vi "Settings Dialog.vi"(8 "error in (no error)":errorcluster, 11 "Settings in":T1) -> (0 "error out":errorcluster, 1 "Cancelled?":bool=TRUE, 2 "UI Refresh Needed?":bool, 3 "Settings out":T5={"Hardware Configuration"={"Analog Out array"=[], "Initialize Flag"=FALSE, "Saftey Table Display"=refnum, "Torque&Force"=[], "Calibration Data"=[], "2D"=[], "Analog In Task"="", "Digital In Task"="", "Analog Out Task"="", "Digital Out Task"="", "Digital Out Array"=[], "Current Cycle Count"=refnum, "Cycle Count"=0, "Headers"=[], "Sweep Interval"=0, "Delay"=0, "TestConfigDisplay"=refnum, "50psi Conversion"=[], "1245N15 Conversion"=[], "MX06F Conversion"=[], "# of Test Cycles"=0, "60psi Conversion"=[], "100psi Conversion"=[], "200psi Conversion"=[], "1000psi Conversion"=[], "2000psi Conversion"=[], "5000psi Conversion"=[], "MX09F Conversion"=[], "MX19F Conversion"=[]}, "Logging Configuration"={"Log File Base Path"=path "C:/Users/jpassiak/Documents/LabVIEW Data/Logged Data.tdms", "TDMS File Reference"=refnum, "Samples to Save"=0, "Trigger - Time"=0, "Trigger - Threshold"=0.0, "Trigger - Channel"=0, "Enable Time Trigger"=FALSE, "Enable Threshold Trigger"=FALSE, "Always Log"=FALSE}, "Configuration Data"={}})   [LabVIEW 2026, in "Settings.lvlib"]
doc: "Dialog for selecting user specified settings."
uses:
  Settings.lvlib
  <vilib>/Utility/xml.llb/Write to XML File(string).vi
  Acquisition/Hardware Configuration.ctl
  Acquisition/Acquisition.lvlib
  Logging/Logging Configuration.ctl
  Logging/Logging.lvlib
  Settings.ctl
  controls/Test Config Data.ctl
panel:
  in  "Log when triggered":bool
  in  "Trigger Channel":u32
  in  "Samples to Log":u32=500 min=1
  in  "Trigger Threshold (V)":dbl=2.0
  in  "Trigger Time (min)":u32=1
  in  "Enable Threshold Trigger (V):":bool
  in  "Enable Time Trigger (min):":bool
  in  "Always Log":bool
  in  "Sample Rate":dbl=1000.0
  in  "Minimum Input":dbl=-10.0
  in  "Maximum Input":dbl=10.0
  in  "DAQmx Channel":tag="Dev1/ai0"
  in  "Log File Path":path
  in  "Cancel Button":bool
  in  "OK Button":bool
  # "Acquisition"
  # "Non visible portion of dialog (needed for connector pane)."
  # "Trigger"
  # "Logging"
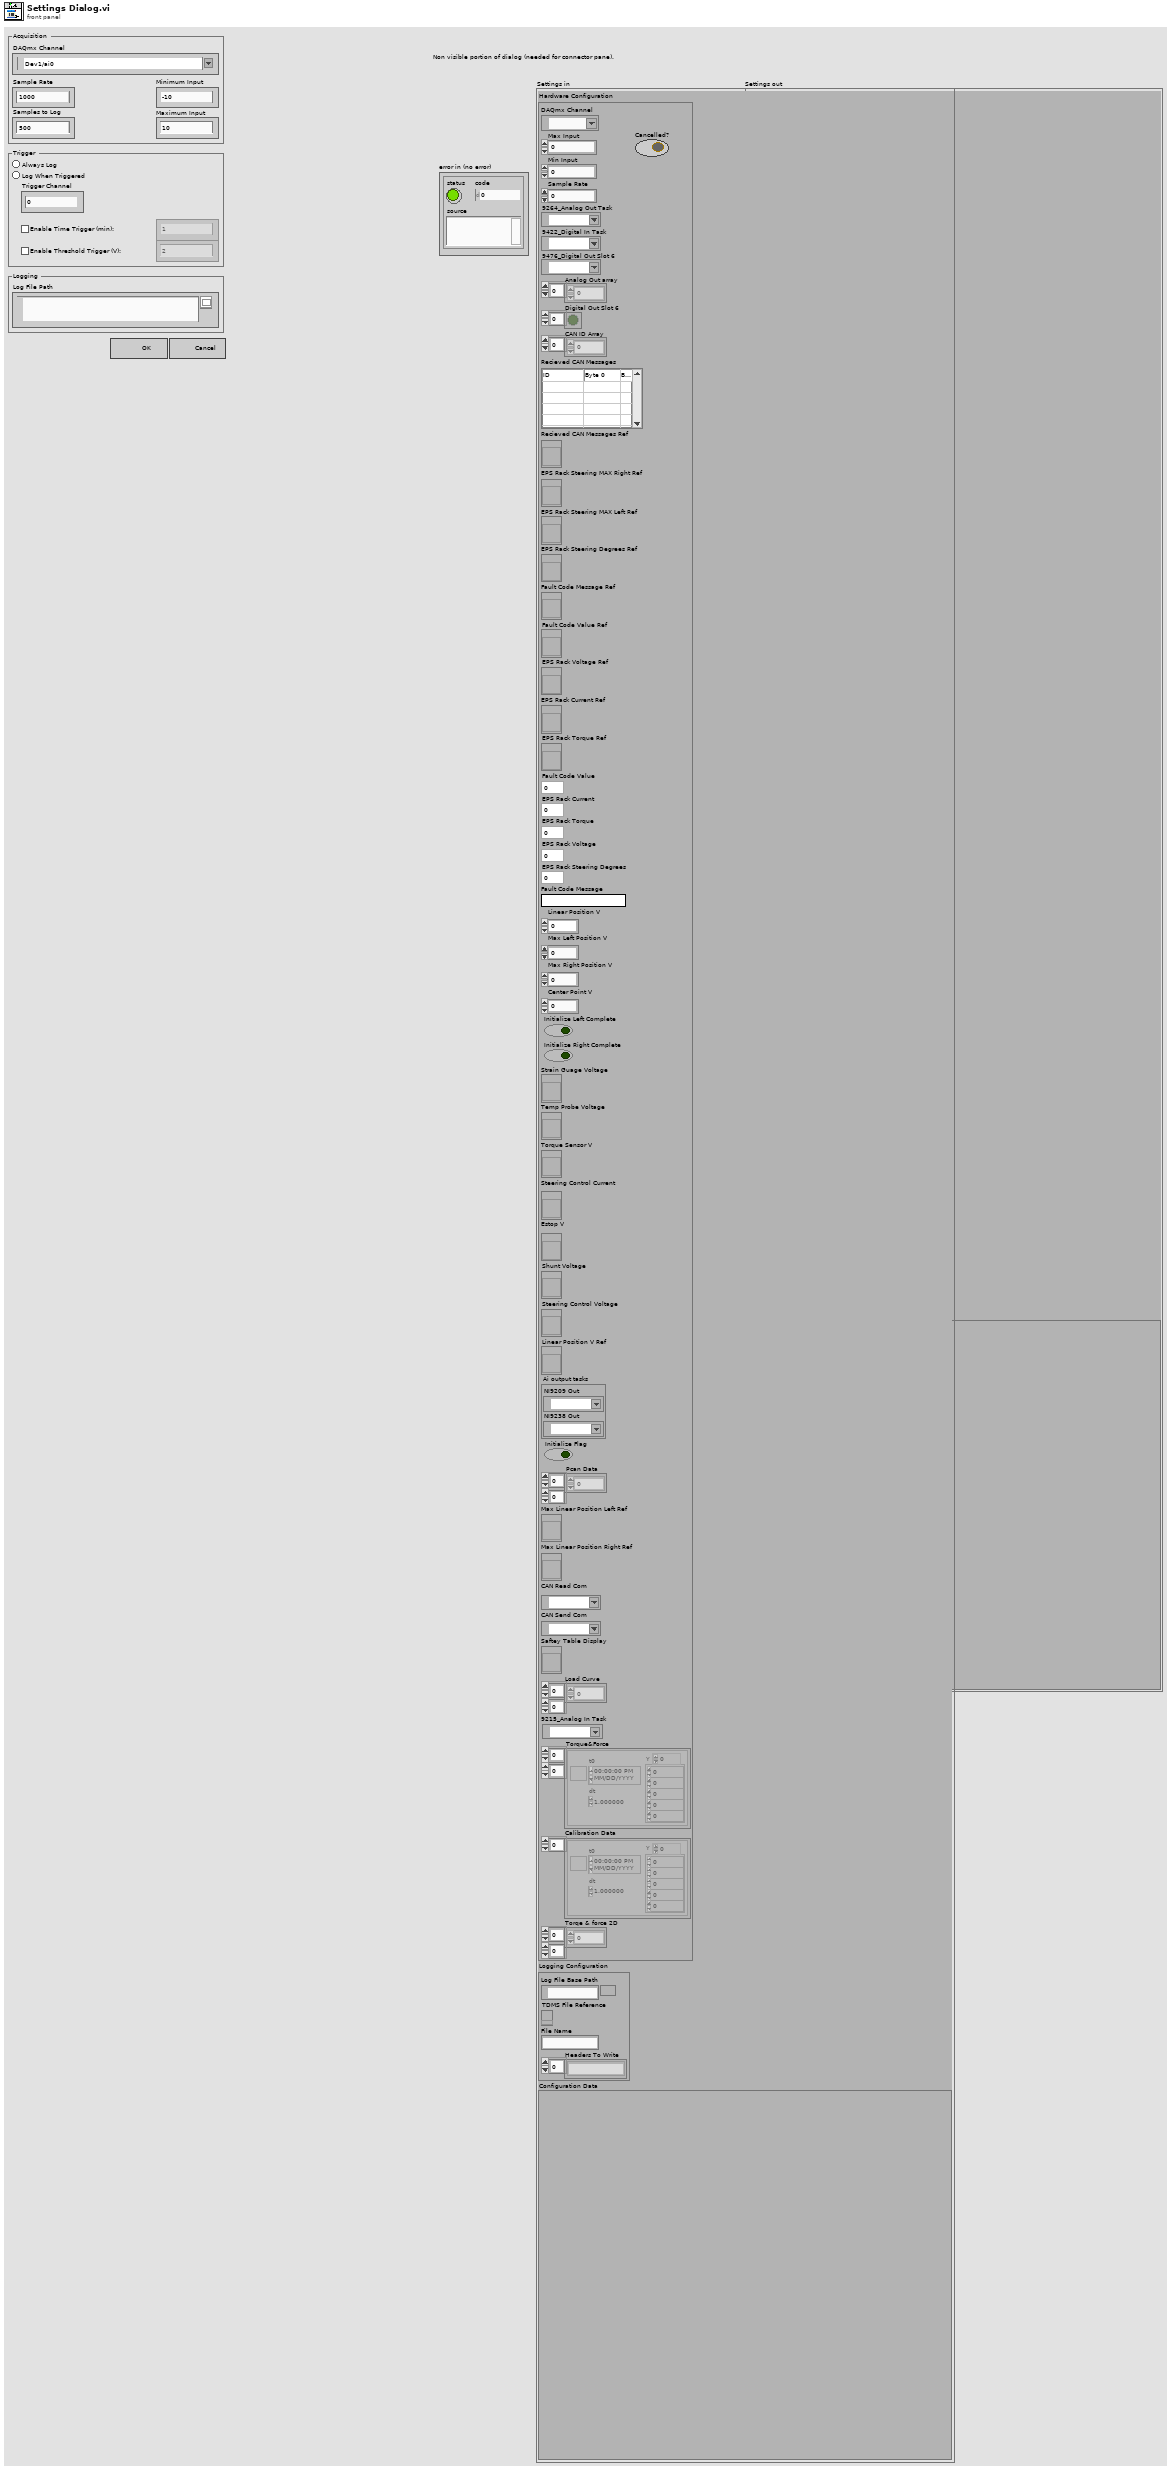
[diagram p1: front panel]
types:
  T1 = typedef "Settings.lvlib/Settings.ctl" = cluster{"Hardware Configuration":T2, "Logging Configuration":T3, "Configuration Data":T4}
  T2 = typedef "Acquisition.lvlib/Hardware Configuration.ctl" = cluster{"DAQmx Channel":tag, "Max Input":dbl, "Min Input":dbl, "Sample Rate":dbl, "9264_Analog Out Task":refnum<k21>, "9422_Digital In Task":refnum<k21>, "9476_Digital Out Slot 6":refnum<k21>, "Analog Out array":dbl[], "Digital Out Slot 6":bool[], "CAN ID Array":u32[], "Recieved CAN Messages ":string[][], "Recieved CAN Messages Ref":refnum<vi>, "EPS Rack Steering MAX Right Ref":refnum<vi>, "EPS Rack Steering MAX Left Ref":refnum<vi>, "EPS Rack Steering Degrees Ref":refnum<vi>, "Fault Code Message Ref":refnum<vi>, "Fault Code Value Ref":refnum<vi>, "EPS Rack Voltage Ref":refnum<vi>, "EPS Rack Current Ref":refnum<vi>, "EPS Rack Torque Ref":refnum<vi>, "Fault Code Value":dbl, "EPS Rack Current":dbl, "EPS Rack Torque":dbl, "EPS Rack Voltage":dbl, "EPS Rack Steering Degrees":dbl, "Fault Code Message":string, "Linear Position V":dbl, "Max Left Position V":dbl, "Max Right Position V":dbl, "Center Point V":dbl, "Initialize Left Complete":bool, "Initialize Right Complete":bool, "Strain Guage Voltage":refnum<vi>, "Temp Probe Voltage":refnum<vi>, "Torque Sensor V":refnum<vi>, "Steering Control Current":refnum<vi>, "Estop V":refnum<vi>, "Shunt Voltage":refnum<vi>, "Steering Control Voltage":refnum<vi>, "Linear Position V Ref":refnum<vi>, "Ai output tasks":cluster{"NI9209 Out":refnum<k21>, "NI9238 Out":refnum<k21>}, "Initialize Flag":bool, "Pcan Data":dbl[][], "Max Linear Position Left Ref":refnum<vi>, "Max Linear Position Right Ref":refnum<vi>, "CAN Read Com":refnum<k21>, "CAN Send Com":refnum<k21>, "Saftey Table Display":refnum<vi>, "Load Curve":dbl[][], "9215_Analog In Task":refnum<k21>, "Torque&Force":waveform(dbl)[][], "Calibration Data":waveform(dbl)[], "Torqe & force 2D":dbl[][]}
  T3 = typedef "Logging.lvlib/Logging Configuration.ctl" = cluster{"Log File Base Path":path, "TDMS File Reference":refnum<k34>, "File Name":string, "Headers To Write":string[]}
  T4 = typedef "Test Config Data.ctl" = cluster{}
  T5 = typedef "Settings.lvlib/Settings.ctl" = cluster{"Hardware Configuration":T6, "Logging Configuration":T7, "Configuration Data":T4}
  T6 = typedef "Acquisition.lvlib/Hardware Configuration.ctl" = cluster{"Analog Out array":dbl[], "Initialize Flag":bool, "Saftey Table Display":refnum<vi>, "Torque&Force":waveform(dbl)[][], "Calibration Data":waveform(dbl)[], "2D":dbl[][], "Analog In Task":refnum<k21>, "Digital In Task":refnum<k21>, "Analog Out Task":refnum<k21>, "Digital Out Task":refnum<k21>, "Digital Out Array":bool[], "Current Cycle Count":refnum<vi>, "Cycle Count":u64, "Headers":string[], "Sweep Interval":u64, "Delay":u64, "TestConfigDisplay":refnum<vi>, "50psi Conversion":dbl[], "1245N15 Conversion":dbl[], "MX06F Conversion":dbl[], "# of Test Cycles":u64, "60psi Conversion":dbl[], "100psi Conversion":dbl[], "200psi Conversion":dbl[], "1000psi Conversion":dbl[], "2000psi Conversion":dbl[], "5000psi Conversion":dbl[], "MX09F Conversion":dbl[], "MX19F Conversion":dbl[]}
  T7 = typedef "Logging.lvlib/Logging Configuration.ctl" = cluster{"Log File Base Path":path, "TDMS File Reference":refnum<k34>, "Samples to Save":u32, "Trigger - Time":u32, "Trigger - Threshold":dbl, "Trigger - Channel":u32, "Enable Time Trigger":bool, "Enable Threshold Trigger":bool, "Always Log":bool}
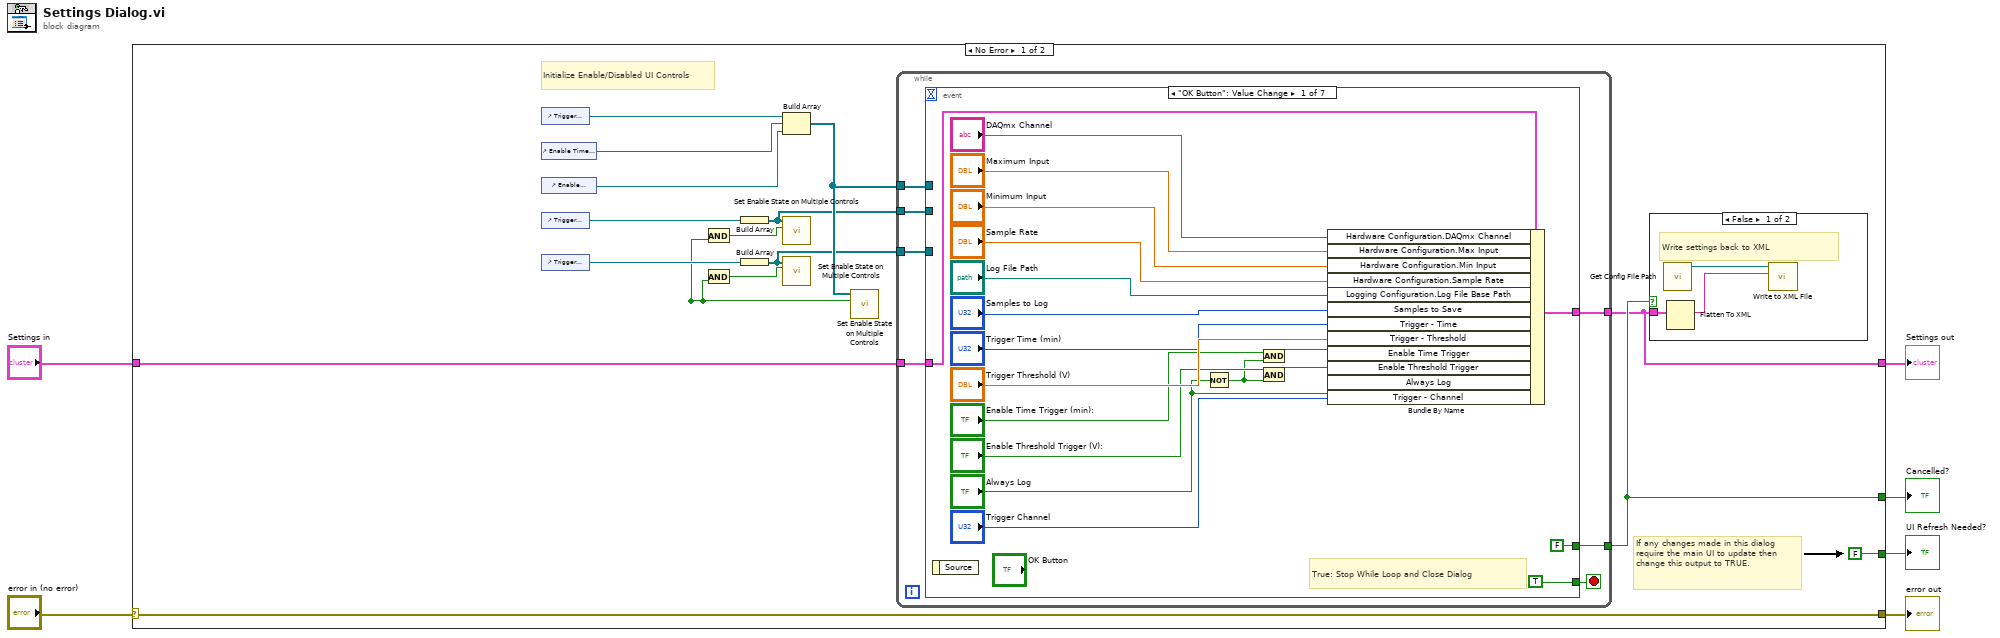
[diagram p0: block diagram]
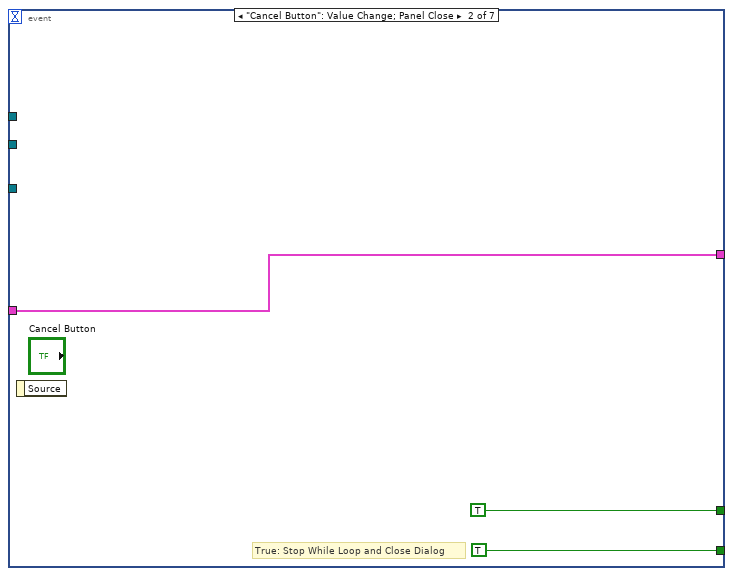
[diagram p2: hidden frame]
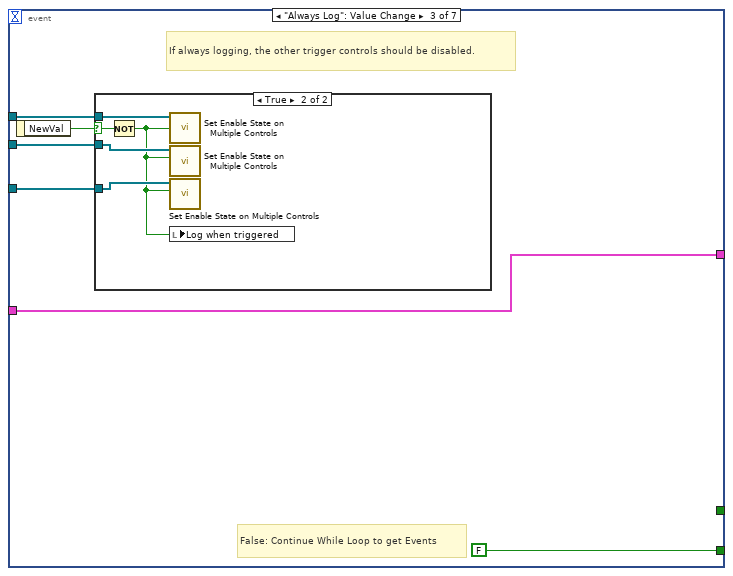
[diagram p3: hidden frame]
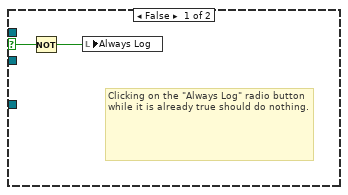
[diagram p4: hidden frame]
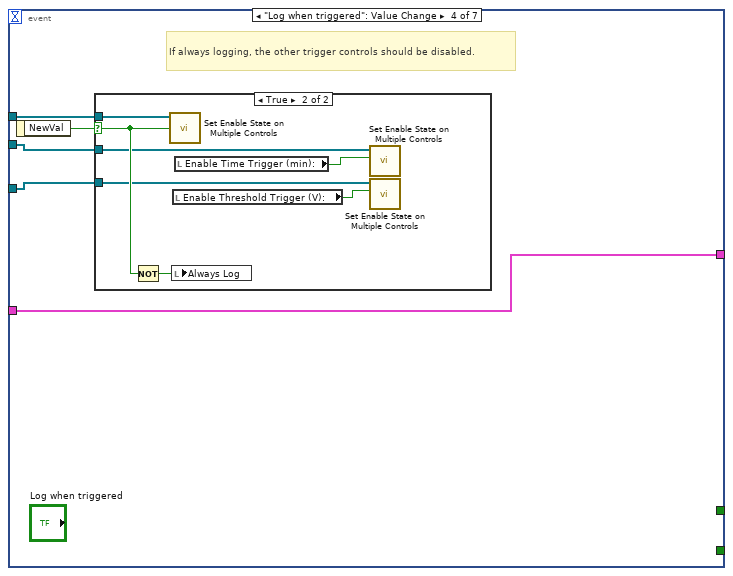
[diagram p5: hidden frame]
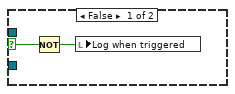
[diagram p6: hidden frame]
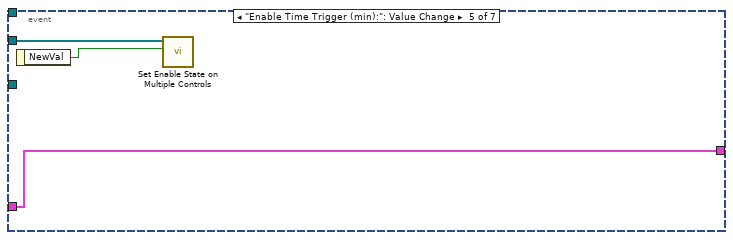
[diagram p7: hidden frame]
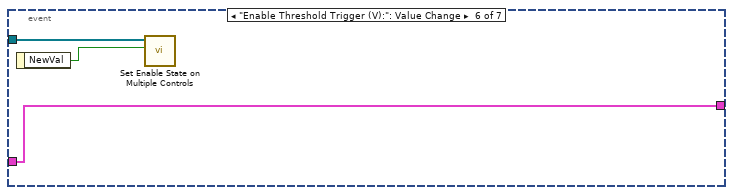
[diagram p8: hidden frame]
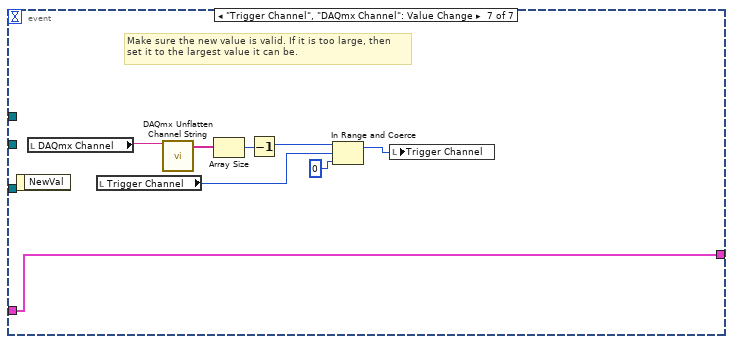
[diagram p9: hidden frame]
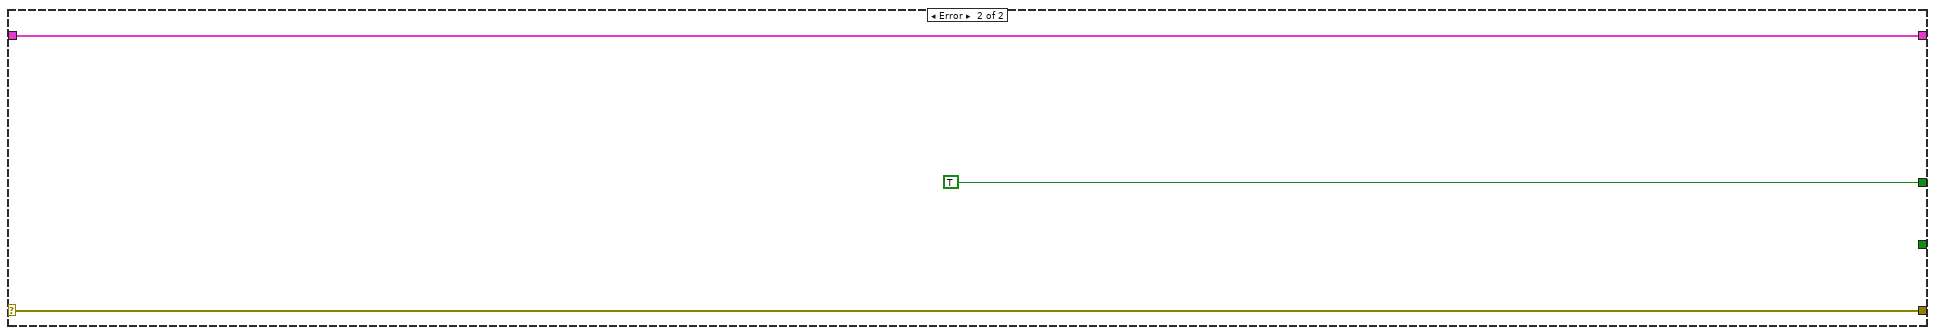
[diagram p11: hidden frame]
diagram:
  n1 = case shown="No Error" "error in (no error)" {
    selector: "error in (no error)" -> [w24 w100]
    tunnel: [w24 w100] -> w6
    tunnel: "Settings in" -> [w19 w99]
    tunnel: [w21 w99] -> w4
    tunnel: [FALSE ("UI Refresh Needed?") _] -> w3
    tunnel: [w22 TRUE ("UI Refresh Needed?")] -> w2
    frame No Error {
      # "Initialize Enable/Disabled UI Controls"
      # "If any changes made in this dialog require the main UI to update then change this output to TRUE."
      n2 = control-ref of="Trigger Channel"() -> (w18:refnum<vi>)
      n3 = control-ref of="Enable Time Trigger (min):"() -> (w17:refnum<vi>)
      n4 = control-ref of="Enable Threshold Trigger (V):"() -> (w16:refnum<vi>)
      n5 = control-ref of="Trigger Time (min)"() -> (w15:refnum<vi>)
      n6 = control-ref of="Trigger Threshold (V)"() -> (w14:refnum<vi>)
      n7 = And() -> (x=w7:bool, y=w8:bool, x .and. y?=w13:bool)
      n8 = And(y=w8) -> (x=w11:bool, x .and. y?=w12:bool)
      n9 = Build Array(w15) -> (w10:refnum<vi>[])
      n10 = Build Array(w14) -> (w9:refnum<vi>[])
      n11 = Build Array(w18, w17, w16) -> (w20:refnum<vi>[])
      n12 = call "Set Enable State on Multiple Controls.vi"("Enable?"=w13, "Controls"=w10) -> ()  [unwired: 10 in]
      n13 = call "Set Enable State on Multiple Controls.vi"("Enable?"=w12, "Controls"=w9) -> ()  [unwired: 10 in]
      n14 = call "Set Enable State on Multiple Controls.vi"("Enable?"=w8, "Controls"=w20) -> ()  [unwired: 10 in]
      n15 = while {
        tunnel: [w31] -> w22
        tunnel: [w30] -> w21
        tunnel: w19 -> [w29]
        tunnel: w20 -> [w27]
        tunnel: w10 -> [w26]
        tunnel: w9 -> [w25]
        stop <- w28 stop-if-true
        n16 = event shown="[0] \"OK Button\": Value Change" {
          selector: _ -> [_ _ _ _ _ _ _]
          dyn-events: _ -> [_ _ _ _ _ _ _]
          timeout: _ -> [_ _ _ _ _ _ _]
          tunnel: [w48 w53 w59 w71 w83 w86 w94] -> w30
          tunnel: w29 -> [w47 w53 w59 w71 w83 w86 w94]
          tunnel: [FALSE ("UI Refresh Needed?") TRUE ("UI Refresh Needed?") _ _ _ _ _] -> w31
          tunnel: [TRUE TRUE FALSE _ _ _ _] -> w28
          tunnel: w27 -> [_ _ w57 w70 _ _ _]
          tunnel: w26 -> [_ _ w55 w68 w82 _ _]
          tunnel: w25 -> [_ _ w54 w67 _ w85 _]
          event "OK Button": Value Change {
            # "True: Stop While Loop and Close Dialog"
            n17 = event-data() -> ()  [unwired: 1 in, 1 out]
            n18 = Not(x="Always Log") -> (.not. x?=w32:bool)
            n19 = And(x="Enable Time Trigger (min):", y=w32) -> (x .and. y?=w33:bool)
            n20 = And(x="Enable Threshold Trigger (V):", y=w32) -> (x .and. y?=w35:bool)
            n21 = Bundle By Name(cluster=w47, "Hardware Configuration.DAQmx Channel"="DAQmx Channel", "Hardware Configuration.Max Input"="Maximum Input", "Hardware Configuration.Min Input"="Minimum Input", "Hardware Configuration.Sample Rate"="Sample Rate", "Logging Configuration.Log File Base Path"="Log File Path", "Samples to Save"="Samples to Log", "Trigger - Time"="Trigger Time (min)", "Trigger - Threshold"="Trigger Threshold (V)", "Enable Time Trigger"=w33, "Enable Threshold Trigger"=w35, "Always Log"="Always Log", "Trigger - Channel"="Trigger Channel") -> (w48:T1)
          }
          event "Cancel Button": Value Change; Panel Close {
            # "True: Stop While Loop and Close Dialog"
            n22 = event-data() -> ()  [unwired: 1 in, 1 out]
          }
          event "Always Log": Value Change {
            # "False: Continue While Loop to get Events"
            # "If always logging, the other trigger controls should be disabled."
            n23 = event-data() -> ("NewVal"=w56:bool)  [unwired: 1 in]
            n24 = case shown="True" w56 {
              selector: w56 -> [w61 w66]
              tunnel: w57 -> [_ w65]
              tunnel: w55 -> [_ w64]
              tunnel: w54 -> [_ w63]
              frame False {
                # "Clicking on the \"Always Log\" radio button while it is already true should do nothing."
                n25 = Not(x=w61) -> (.not. x?=w60:bool)
                n26 = local write "Always Log"(w60) -> ()
              }
              frame True {
                n27 = Not(x=w66) -> (.not. x?=w62:bool)
                n28 = call "Set Enable State on Multiple Controls.vi"("Enable?"=w62, "Controls"=w65) -> ()  [unwired: 10 in]
                n29 = call "Set Enable State on Multiple Controls.vi"("Enable?"=w62, "Controls"=w64) -> ()  [unwired: 10 in]
                n30 = call "Set Enable State on Multiple Controls.vi"("Enable?"=w62, "Controls"=w63) -> ()  [unwired: 10 in]
                n31 = local write "Log when triggered"(w62) -> ()
              }
            }
          }
          event "Log when triggered": Value Change {
            # "If always logging, the other trigger controls should be disabled."
            n32 = event-data() -> ("NewVal"=w69:bool)  [unwired: 1 in]
            n33 = case shown="True" w69 {
              selector: w69 -> [w73 w79]
              tunnel: w70 -> [_ w80]
              tunnel: w68 -> [_ w77]
              tunnel: w67 -> [_ w76]
              frame False {
                n34 = Not(x=w73) -> (.not. x?=w72:bool)
                n35 = local write "Log when triggered"(w72) -> ()
              }
              frame True {
                n36 = Not(x=w79) -> (.not. x?=w78:bool)
                n37 = call "Set Enable State on Multiple Controls.vi"("Enable?"=w79, "Controls"=w80) -> ()  [unwired: 10 in]
                n38 = local write "Always Log"(w78) -> ()
                n39 = local read "Enable Threshold Trigger (V):"() -> (w75:bool)
                n40 = local read "Enable Time Trigger (min):"() -> (w74:bool)
                n41 = call "Set Enable State on Multiple Controls.vi"("Enable?"=w74, "Controls"=w77) -> ()  [unwired: 10 in]
                n42 = call "Set Enable State on Multiple Controls.vi"("Enable?"=w75, "Controls"=w76) -> ()  [unwired: 10 in]
              }
            }
          }
          event "Enable Time Trigger (min):": Value Change {
            n43 = event-data() -> ("NewVal"=w81:bool)  [unwired: 1 in]
            n44 = call "Set Enable State on Multiple Controls.vi"("Enable?"=w81, "Controls"=w82) -> ()  [unwired: 10 in]
          }
          event "Enable Threshold Trigger (V):": Value Change {
            n45 = event-data() -> ("NewVal"=w84:bool)  [unwired: 1 in]
            n46 = call "Set Enable State on Multiple Controls.vi"("Enable?"=w84, "Controls"=w85) -> ()  [unwired: 10 in]
          }
          event "Trigger Channel", "DAQmx Channel": Value Change {
            # "Make sure the new value is valid. If it is too large, then\nset it to the largest value it can be."
            n47 = event-data() -> ()  [unwired: 1 in, 1 out]
            n48 = local read "DAQmx Channel"() -> (w93:tag)
            n49 = local read "Trigger Channel"() -> (w87:u32)
            n50 = call <vilib>:"DAQmx Unflatten Channel String.vi"("names in"=w93) -> ("names out"=w92:string[])  [unwired: 13 in, 1 out]
            n51 = Array Size(array=w92) -> (size(s)=w91:i32)
            n52 = Decrement(x=w91) -> (x-1=w90:i32)
            n53 = In Range and Coerce(upper limit=w90, x=w87, lower limit=u32 0) -> (coerced(x)=w88:u32)  [unwired: 1 out]
            n54 = local write "Trigger Channel"(w88) -> ()
          }
        }
      }
      n55 = case shown="False" w22 {
        tunnel: w21 -> [w96 _]
        frame False {
          # "Write settings back to XML"
          n56 = call "Get Config File Path.vi"() -> ("XML File Path"=w97:path)  [unwired: 10 in, 1 out]
          n57 = Flatten To XML(6:w96) -> (2:w95:string)
          n58 = call-poly <vilib>:"Write to XML File.vi"("XML Input"=w95, "XML File Path"=w97) -> ()  [unwired: 7 in, 3 out]
        }
        frame True {
        }
      }
    }
    frame Error {
    }
  }
  "UI Refresh Needed?" <- w3
  "error out" <- w6
  "Settings out" <- w4
  "Cancelled?" <- w2
